vi "Autotest_Instr.vi"(8 "error in (no error)":errorcluster caption="entrée d'erreur (pas d'erreur)", 11 "Class Instrument Multimeter en entrée":refnum<class "Class Instrument Multimeter.lvclass">) -> (0 "error out":errorcluster caption="sortie d'erreur", 3 "Class Instrument Multimeter en sortie":refnum<class "Class Instrument Multimeter.lvclass">)   [LabVIEW 2020, in "Library Instrument & Equipement.lvlib" / "Library Instruments.lvlib" / "Class Instrument Multimeter.lvclass"]
uses:
  Class Instrument Multimeter.lvclass
  C:/Users/ngarcin/OneDrive - Altyor/Standard TB/Class/Instrument/Instrument (Default)/Class Instrument (Default).lvclass
  Class Instrument Multimeter.lvclass/Class Instrument Multimeter.ctl
  Instrument (Default)/Class Instrument (Default).lvclass
  Multimeter/Multimeter (Default)/Class Multimeter (Default).lvclass
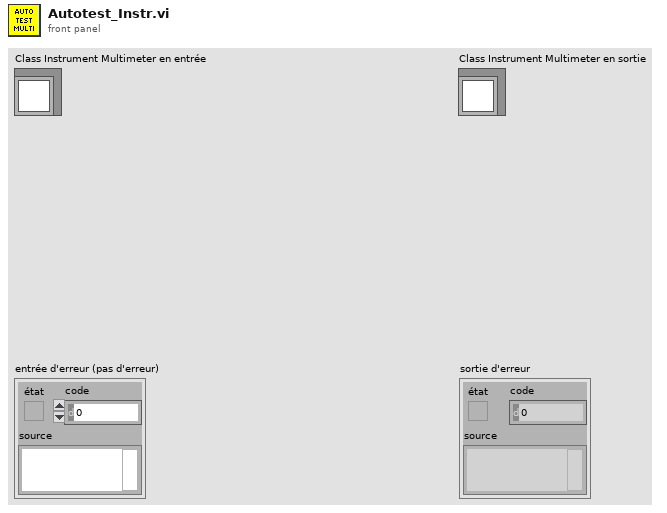
[diagram p1: front panel]
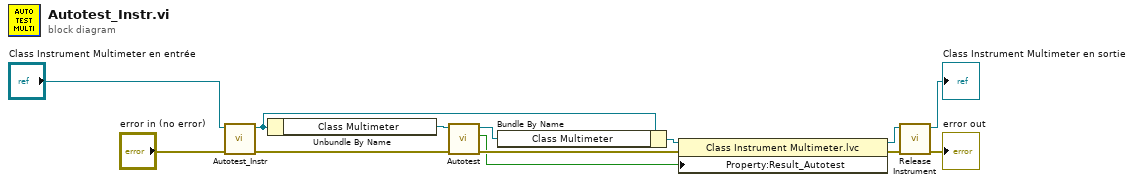
[diagram p0: block diagram]
diagram:
  n1 = call-parent "Autotest_Instr.vi"("error in (no error)"="error in (no error)", "Class Instrument (Default) en entrée"="Class Instrument Multimeter en entrée") -> ("error out"=w10:errorcluster, "Class Instrument (Default) en sortie"=w8:refnum<class "Class Instrument Multimeter.lvclass">)  [unwired: 8 in]
  n2 = Unbundle By Name(w8) -> ("Class Multimeter"=w11:refnum<class "Class Multimeter (Default).lvclass">)
  n3 = call-dynamic "Autotest.vi"("error in (no error)"=w10, "Class Multimeter (Default) en entrée"=w11) -> ("error out"=w7:errorcluster, "Autotest Ok ?"=w5:bool, "Class Multimeter (Default) en sortie"=w9:refnum<class "Class Multimeter (Default).lvclass">)  [unwired: 7 in]
  n4 = Bundle By Name(cluster=w8, "Class Multimeter"=w9) -> (w6:refnum<class "Class Instrument Multimeter.lvclass">)
  n5 = property class="Class Instrument Multimeter.lvc"(reference=w6, error in=w7, "Property:Result_Autotest"=w5) -> (reference out=w2:refnum<class "Class Instrument Multimeter.lvclass">, error out=w4:errorcluster)
  n6 = call-dynamic "Release Instrument.vi"("error in (no error)"=w4, "Class Instrument (Default) en entrée"=w2) -> ("error out"=→"error out":errorcluster, "Class Instrument (Default) en sortie"=→"Class Instrument Multimeter en sortie":refnum<class "Class Instrument Multimeter.lvclass">)  [unwired: 8 in]
